vi "Illini Hyperloop GUI v3.2.vi"() -> ()   [LabVIEW 2015]
uses:
  <vilib>/robotics/Controls/Attitude Indicator/Attitude Indicator.xctl
  CommunicationStatus.ctl
  StageEnum.ctl
  BlockDiagramControlEnum.ctl
panel:
  out "Braking Force":dbl
  out "Braking Force Chart":dbl(slide) caption="Braking Force (N)" scale=0.0..10000.0
  out "Current 6":dbl[unit] caption="Current"
  out "Voltage 6":dbl[unit] caption="Voltage"
  out "RPM 6":dbl[unit] caption="RPM"
  out "Current 5":dbl[unit] caption="Current"
  out "Voltage 5":dbl[unit] caption="Voltage"
  out "RPM 5":dbl[unit] caption="RPM"
  out "Current 4":dbl[unit] caption="Current"
  out "Voltage 4":dbl[unit] caption="Voltage"
  out "RPM 4":dbl[unit] caption="RPM"
  out "Current 3":dbl[unit] caption="Current"
  out "Voltage 3":dbl[unit] caption="Voltage"
  out "RPM 3":dbl[unit] caption="RPM"
  out "Current 2":dbl[unit] caption="Current"
  out "Voltage 2":dbl[unit] caption="Voltage"
  out "RPM 2":dbl[unit] caption="RPM"
  out "Current 1":dbl[unit] caption="Current"
  out "Voltage 1":dbl[unit] caption="Voltage"
  out "RPM 1":dbl[unit] caption="RPM"
  out "Flight Time":string
  out "Attitude Indicator":cluster{"Roll":dbl, "Pitch":dbl}(xcontrol)
  out "Yaw":dbl(knob) scale=-20.0..20.0
  out "RPM Gauge 6":dbl(knob) scale=0.0..2000.0
  out "RPM Gauge 5":dbl(knob) scale=0.0..2000.0
  out "RPM Gauge 4":dbl(knob) scale=0.0..2000.0
  out "RPM Gauge 3":dbl(knob) scale=0.0..2000.0
  out "RPM Gauge 2":dbl(knob) scale=0.0..2000.0
  out "RPM Gauge 1":dbl(knob) scale=0.0..2000.0
  out "Cabin Pressure":dbl format="%#.3g"
  out "Cabin Pressure (psi)":dbl(graph)
  out "Stage":T1
  out "Communication Status":T2
  out "Levitation Height":dbl[unit]
  out "Computing:":dbl format="%#.2g"
  out "Low Battery":dbl format="%#.2g"
  out "High Battery:":dbl format="%#.2g"
  out "Battery 3":dbl(slide) scale=0.0..100.0
  out "Battery 2":dbl(slide) scale=0.0..100.0
  out "Battery 1":dbl(slide) scale=0.0..100.0
  out "Z acceleration":dbl
  out "Y acceleration":dbl
  out "X acceleration":dbl
  out "Z velocity":dbl
  out "Y velocity":dbl
  out "X velocity":dbl
  out "Z position":dbl
  out "Y position":dbl
  out "X position":dbl
  out "Position (m)":dbl(slide) scale=0.0..2490.0
  out "Velocity (m/s)":dbl(graph)
  in  "EMERGENCY BRAKE":bool
  in  "Functional Test Tab Control":T3(tab)
  out "Functional Test A Data":string caption="Data:"
  in  "Functional Test 1":bool caption="Boolean"
  out "Functional Test B Data":string caption="Data:"
  in  "Functional Test 2":bool caption="Boolean"
  out "Functional Test C Data":string caption="Data:"
  in  "Functional Test 3":bool caption="Boolean"
  in  "Functional Test 4":bool caption="Boolean"
  out "Functional Test D Data":string caption="Data:"
  out "Client Closed":string="The client VI closed the connection."
  out "Data out":string
  out "remote address":string
  out "remote port":u16
  in  "Connect to":string="192.168.137.10"
  in  "timeout ms":i32=25000
  in  "port":u16=5005
  in  "Prepare for Launch":bool caption="Boolean"
  in  "Stop Program":bool
  out "Error Messages":errorcluster
  out "Temp 2:":dbl format="%.2g"
  out "Temp 1:":dbl format="%.2g"
  out "Temperature (K)":dbl[](graph)
  out "Acceleration Chart":dbl(graph)
  out "Checkmark":u16(ring)
  # "Illini Hyperloop"
  # "Arx Pax"
  # "Front"
  # "Attitude"
  # "Acceleration (m/s/s)"
  # "Battery Levels (%)"
  # "More battery?????"
  # "Functional Test A: Power Up and Communication"
  # "Functional Test B: Levitation"
  # "Functional Test C: Communication Inside Tube"
  # "Functional Test D: Internal power and Levitation"
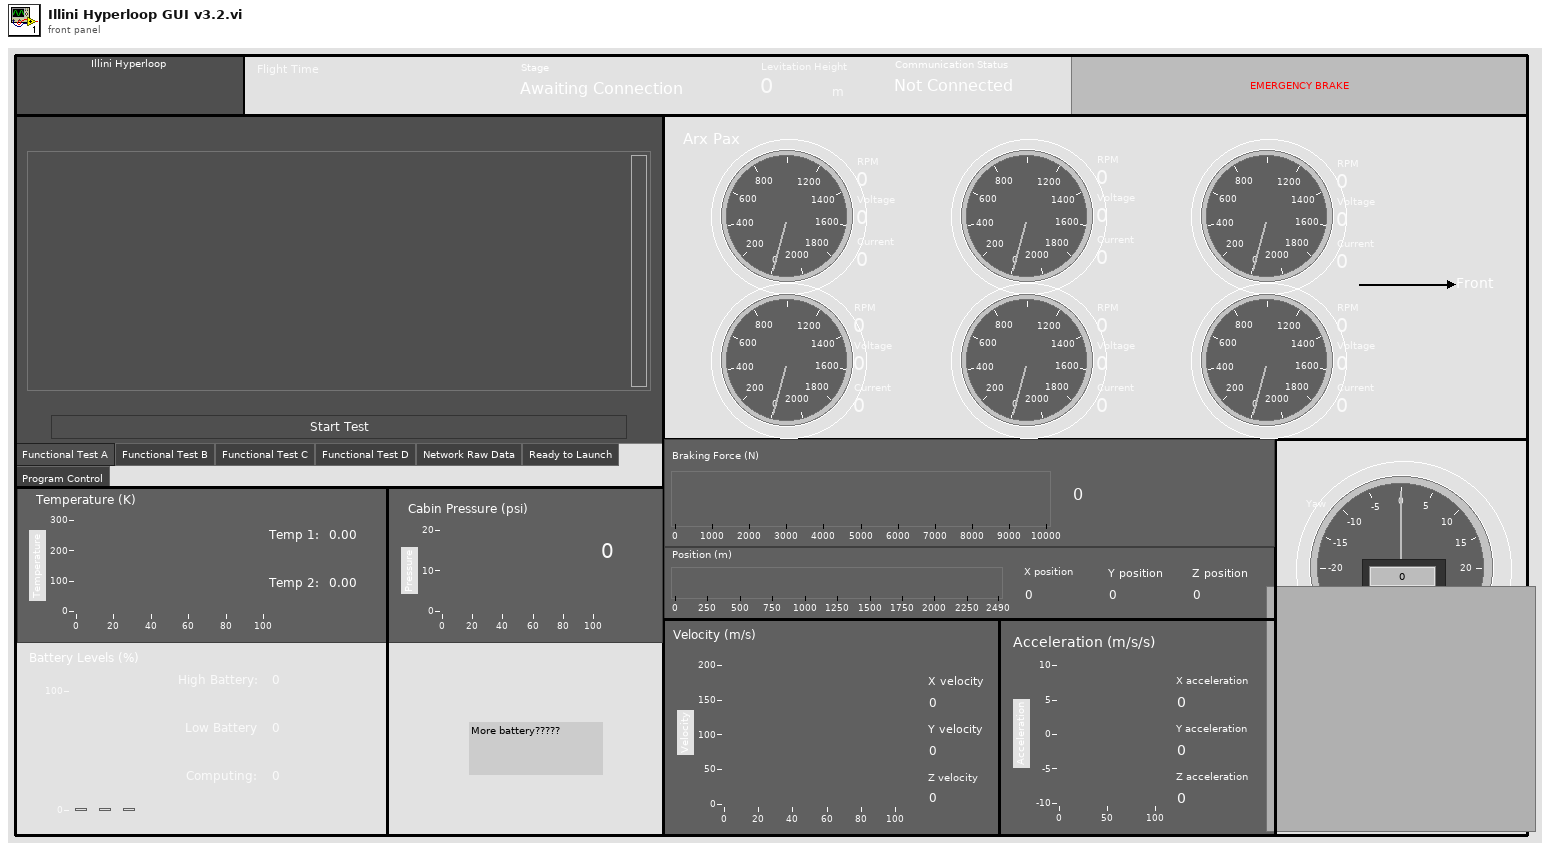
[diagram p1: front panel]
types:
  T1 = typedef "StageEnum.ctl" = enum16{"Awaiting Connection", "TEST Comms", "TEST Lev", "TEST Inside Comms", "TEST Internal Power", "Ready to Launch", "Acceleration", "Coast", "Brake"}
  T2 = typedef "CommunicationStatus.ctl" = enum16{"Not Connected", "Connected", "Disconnected"}
  T3 = enum32{"Functional Test A", "Functional Test B", "Functional Test C", "Functional Test D", "Network Raw Data", "Ready to Launch", "Program Control"}
  T4 = typedef "BlockDiagramControlEnum.ctl" = enum16{"Not Connected", "Disconnected", "Functional Test A", "Functional Test B", "Functional Test C", "Functional Test D", "Flight"}
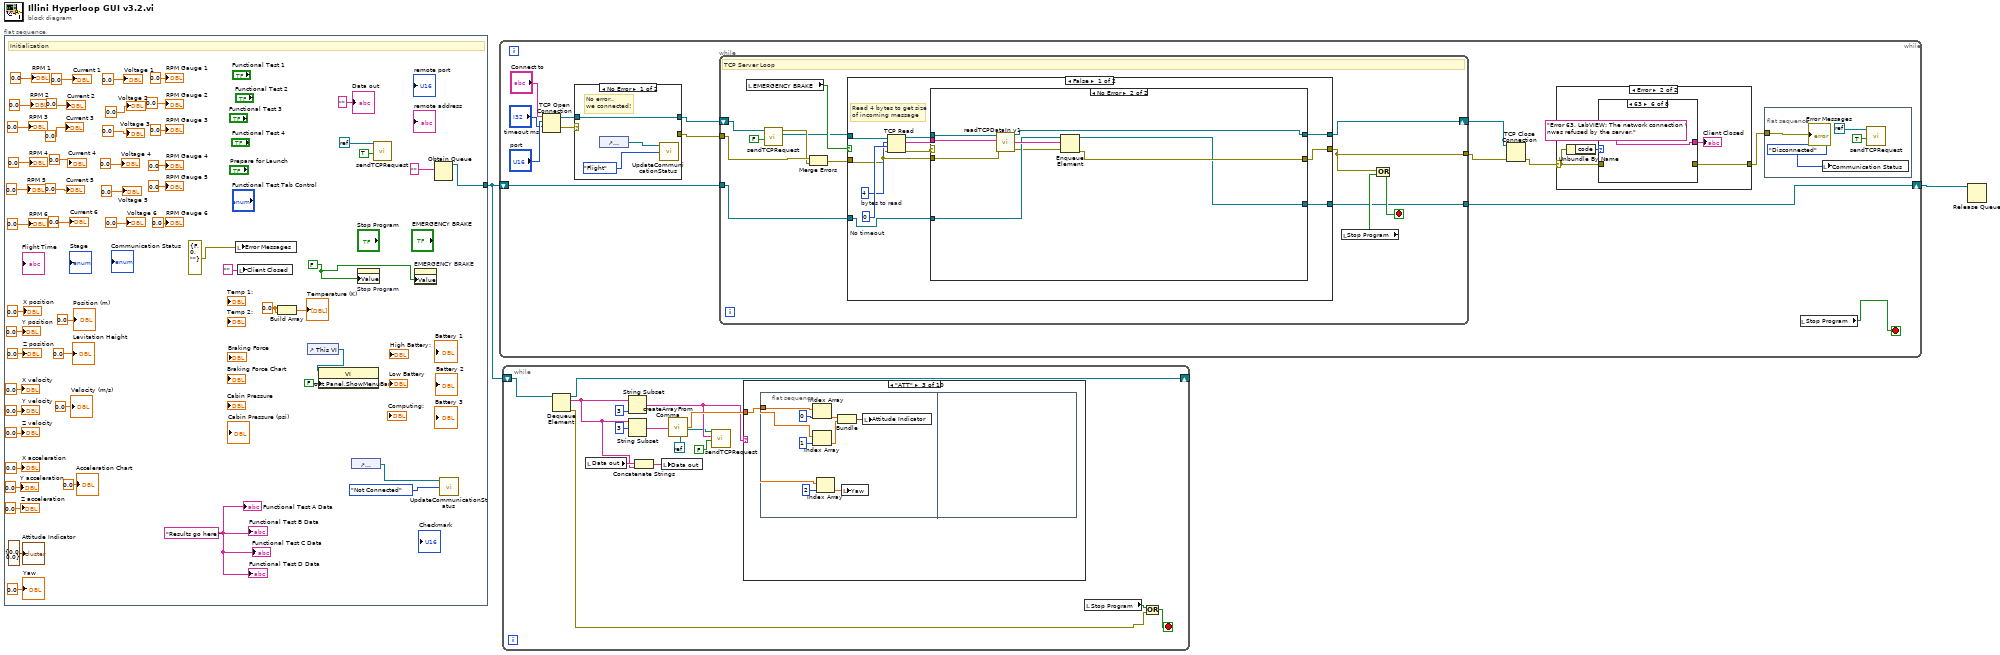
[diagram p0: block diagram]
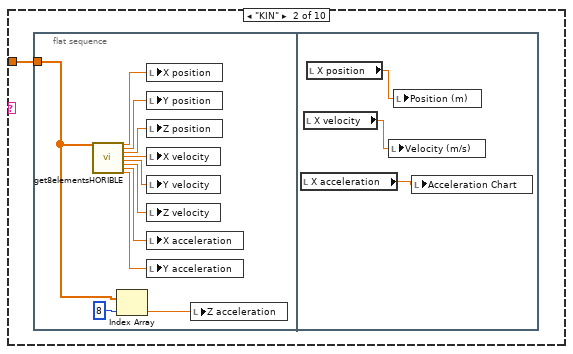
[diagram p3: hidden frame]
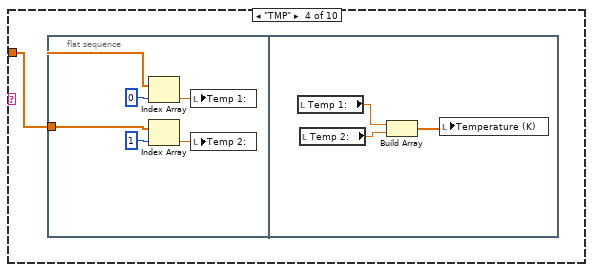
[diagram p4: hidden frame]
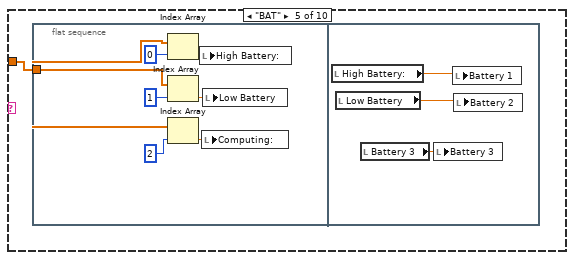
[diagram p5: hidden frame]
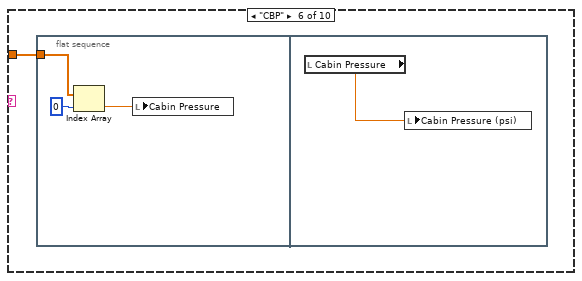
[diagram p6: hidden frame]
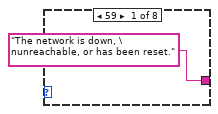
[diagram p13: hidden frame]
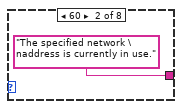
[diagram p14: hidden frame]
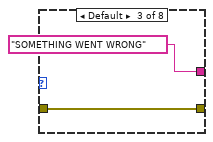
[diagram p15: hidden frame]
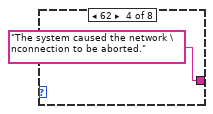
[diagram p16: hidden frame]
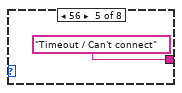
[diagram p17: hidden frame]
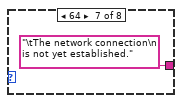
[diagram p18: hidden frame]
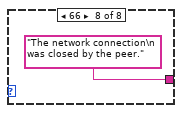
[diagram p19: hidden frame]
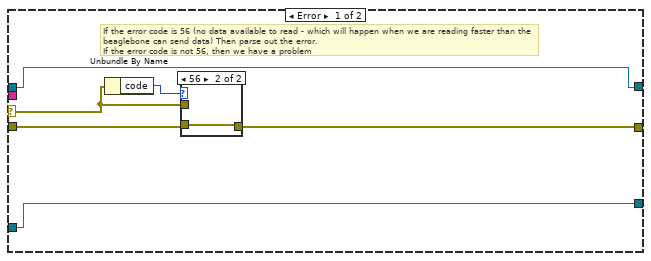
[diagram p20: hidden frame]
diagram:
  n1 = flat-sequence {
    tunnel: [w54] -> w2
    frame #0 {
      w9 = FALSE
      w14 = "Results go here!" ("Functional Test 1 Data")
      w29 = 0.0 ("element")
      # "Initialization"
      n2 = local write "Error Messages"(errorcluster {"status"=FALSE, "code"=0, "source"=""} ("error constant")) -> ()
      n3 = local write "Client Closed"("" ("Client Closed")) -> ()
      n4 = Build Array(w29, w29) -> (→"Temperature (K)":dbl[])
      n5 = control-ref of="This VI"() -> (w8:refnum<vi>)
      n6 = property class="VI"(reference=w8, "Front Panel.ShowMenuBar"=FALSE ("Front Panel Window:Show Menu Bar")) -> ()  [unwired: 1 in, 2 out]
      n7 = control-ref of="Communication Status"() -> (w56:refnum<vi>)
      n8 = property on="Stop Program" class="Bool (strict)"("Value"=w9) -> ()  [unwired: 2 in, 2 out]
      n9 = call "sendTCPRequest.vi"("Force Reset"=TRUE, "TCP Network Connection in"=refnum<k0> refnum) -> ()  [unwired: 8 in, 2 out]
      n10 = property on="EMERGENCY BRAKE" class="Bool (strict)"("Value"=w9) -> ()  [unwired: 2 in, 2 out]
      n11 = Obtain Queue(element data type="") -> (queue out=w54:refnum<queue>)  [unwired: 4 in, 2 out]
      n12 = call "UpdateCommunicationStatus.vi"("Block Diagram Control Enum"=BlockDiagramControlEnum."Not Connected", "Communication Enum Refnum in"=w56) -> ()  [unwired: 1 in]
      "RPM Gauge 2" <- 0.0 ("RPM Gauge 2")
      "RPM Gauge 4" <- 0.0 ("RPM Gauge 4")
      "RPM Gauge 5" <- 0.0 ("RPM Gauge 5")
      "RPM Gauge 1" <- 0.0 ("RPM Gauge 1")
      "RPM Gauge 6" <- 0.0 ("RPM Gauge 6")
      "RPM Gauge 3" <- 0.0 ("RPM Gauge 3")
      "RPM 1" <- dbl[unit] 0.0 ("RPM 1")
      "Current 1" <- dbl[unit] 0.0 ("Current 1")
      "RPM 2" <- dbl[unit] 0.0 ("RPM 2")
      "Voltage 2" <- dbl[unit] 0.0 ("Voltage 2")
      "Current 2" <- dbl[unit] 0.0 ("Current 2")
      "RPM 3" <- dbl[unit] 0.0 ("RPM 3")
      "Voltage 3" <- dbl[unit] 0.0 ("Voltage 3")
      "Current 3" <- dbl[unit] 0.0 ("Current 3")
      "RPM 4" <- dbl[unit] 0.0 ("RPM 4")
      "Voltage 4" <- dbl[unit] 0.0 ("Voltage 4")
      "Current 4" <- dbl[unit] 0.0 ("Current 4")
      "RPM 5" <- dbl[unit] 0.0 ("RPM 5")
      "Voltage 5" <- dbl[unit] 0.0 ("Voltage 5")
      "Current 5" <- dbl[unit] 0.0 ("Current 5")
      "RPM 6" <- dbl[unit] 0.0 ("RPM 6")
      "Voltage 6" <- dbl[unit] 0.0 ("Voltage 6")
      "Current 6" <- dbl[unit] 0.0 ("Current 6")
      "Voltage 1" <- dbl[unit] 0.0 ("Voltage 1")
      "Position (m)" <- 0.0 ("Position (m)")
      "X position" <- 0.0 ("X position")
      "Y position" <- 0.0 ("Y position")
      "Z position" <- 0.0 ("Z position")
      "X velocity" <- 0.0 ("X velocity")
      "Y velocity" <- 0.0 ("Y velocity")
      "Z velocity" <- 0.0 ("Z velocity")
      "X acceleration" <- 0.0 ("X acceleration")
      "Y acceleration" <- 0.0 ("Y acceleration")
      "Z acceleration" <- 0.0 ("Z acceleration")
      "Velocity (m/s)" <- 0.0 ("Velocity (m/s)")
      "Attitude Indicator" <- cluster{"Roll":dbl, "Pitch":dbl} {"Roll"=0.0, "Pitch"=0.0} ("Attitude Indicator")
      "Levitation Height" <- dbl[unit] 0.0 ("Levitation Height")
      "Acceleration Chart" <- 0.0 ("Acceleration Chart")
      "Yaw" <- 0.0 ("Yaw")
      "Functional Test A Data" <- w14
      "Functional Test B Data" <- w14
      "Functional Test C Data" <- w14
      "Functional Test D Data" <- w14
      "Data out" <- "" ("Data out")
    }
  }
  n13 = while {
    shift-right: [w63] -> w1
    shift-left: w2 -> [w64]
    stop <- w60 stop-if-true
    n14 = TCP Open Connection(address="Connect to", remote port or service name="port", timeout ms (60000)="timeout ms") -> (connection ID=w65:refnum<k5>, error out=w66:errorcluster)  [unwired: 2 in]
    n15 = case shown="No Error" w66 {
      selector: w66 -> [_ w78]
      tunnel: w65 -> [w77 w79]
      tunnel: [w77 w79] -> w58
      tunnel: [_ w78] -> w57
      frame No Error {
        # "No error.. \nwe connected!"
        n16 = control-ref of="Communication Status"() -> (w76:refnum<vi>)
        n17 = call "UpdateCommunicationStatus.vi"("Block Diagram Control Enum"=BlockDiagramControlEnum."Flight", "Communication Enum Refnum in"=w76) -> ()  [unwired: 1 in]
      }
      frame Error {
      }
    }
    n18 = while {
      tunnel: w57 -> [w98]
      tunnel: [w104] -> w62
      tunnel: w64 -> [w102]
      tunnel: [w101] -> w63
      shift-right: [w100] -> w59
      shift-left: w58 -> [w99]
      stop <- w103 stop-if-true
      # "TCP Server Loop"
      n19 = local read "EMERGENCY BRAKE"() -> (w106:bool)
      n20 = call "sendTCPRequest.vi"("Force Reset"=FALSE, "TCP Network Connection in"=w99) -> ("Connection Out"=w96:refnum<k5>, "error out"=w97:errorcluster)  [unwired: 8 in]
      n21 = Merge Errors(w98, w97) -> (w94:errorcluster)
      n22 = case shown="False" w106 {
        tunnel: w94 -> [w115 w140]
        tunnel: w96 -> [w116 w139]
        tunnel: [w112 w138] -> w100
        tunnel: [w108 w137] -> w104
        tunnel: w102 -> [w110 w136]
        tunnel: [w109 w136] -> w101
        frame False {
          w117 = 4  # bytes to read
          w118 = 0  # No timeout
          # "Read 4 bytes to get size\nof incoming message"
          n23 = TCP Read(connection ID=w116, bytes to read=w117, error in (no error)=w115, 9:w118) -> (connection ID out=w113:refnum<k5>, data out=w111:string, error out=w114:errorcluster)  [unwired: 1 in]
          n24 = case shown="No Error" w114 {
            selector: w114 -> [w122 _]
            tunnel: w115 -> [w123 w133]
            tunnel: [w121 w128] -> w108
            tunnel: w113 -> [w120 w134]
            tunnel: [w120 w132] -> w112
            tunnel: w111 -> [_ w135]
            tunnel: w110 -> [w119 w130]
            tunnel: [w119 w127] -> w109
            frame Error {
              # "If the error code is 56 (no data available to read - which will happen when we are reading faster than the beaglebone can send data) Then parse out the error. \nIf the error code is not 56, then we have a problem"
              n25 = Unbundle By Name(w122) -> ("code"=w124:i32)
              n26 = case shown="56" w124 {
                tunnel: w122 -> [w125 _]
                tunnel: [w125 w126] -> w121
                tunnel: w123 -> [_ w126]
                frame Default {
                }
                frame 56 {
                }
              }
            }
            frame No Error {
              n27 = call "readTCPDataIn v1.vi"("TCP Network Connection in"=w134, "Size of data"=w135, "error in (no error)"=w133) -> ("TCP Network Connection out"=w132:refnum<k5>, "Operation+Data"=w131:string, "error out"=w129:errorcluster)  [unwired: 8 in, 2 out]
              n28 = Enqueue Element(queue=w130, element=w131, error in (no error)=w129) -> (queue out=w127:refnum<queue>, error out=w128:errorcluster)  [unwired: 1 in, 1 out]
            }
          }
        }
        frame True {
          n29 = TCP Write(connection ID=w139, data in="STOP!STOP", error in (no error)=w140) -> (connection ID out=w138:refnum<k5>, error out=w137:errorcluster)  [unwired: 1 in, 1 out]
        }
      }
      n30 = local read "Stop Program"() -> (w105:bool)
      n31 = Or(x=w104, y=w105) -> (x .or. y?=w103:bool)
      n32 = Wait (ms)(milliseconds to wait=u32 0) -> ()  [unwired: 1 out]
    }
    n33 = TCP Close Connection(connection ID=w59, error in (no error)=w62) -> (error out=w70:errorcluster)  [unwired: 2 out]
    n34 = case shown="Error" w70 {
      selector: w70 -> [w80 w83]
      tunnel: [w80 w82] -> w69
      frame No Error {
      }
      frame Error {
        n35 = Unbundle By Name(w83) -> ("code"=w84:i32)
        n36 = case shown="63" w84 {
          tunnel: w83 -> [_ _ w88 _ _ _ _ _]
          tunnel: [_ _ w88 _ _ _ _ _] -> w82
          tunnel: ["The network is down, \nunreachable, or has been reset." "The specified network \naddress is currently in use." "SOMETHING WENT WRONG" "The system caused the network \nconnection to be aborted." "Timeout / Can't connect" "Error 63. LabVIEW: The network connection \nwas refused by the server." "\tThe network connection\n is not yet established." "The network connection\n was closed by the peer."] -> w81
          frame 59 {
          }
          frame 60 {
          }
          frame Default {
          }
          frame 62 {
          }
          frame 56 {
          }
          frame 63 {
          }
          frame 64 {
          }
          frame 66 {
          }
        }
        "Client Closed" <- w81
      }
    }
    n37 = flat-sequence {
      tunnel: w69 -> [w74]
      frame #0 {
        n38 = local write "Communication Status"(CommunicationStatus."Disconnected" ("Communication Status")) -> ()
        n39 = call "sendTCPRequest.vi"("Force Reset"=TRUE, "TCP Network Connection in"=refnum<k0> refnum) -> ()  [unwired: 8 in, 2 out]
        "Error Messages" <- w74
      }
    }
    n40 = local read "Stop Program"() -> (w60:bool)
  }
  n41 = while {
    shift-right: [w156] -> _
    shift-left: w2 -> [w151]
    stop <- w145 stop-if-true
    n42 = Dequeue Element(queue=w151) -> (queue out=w156:refnum<queue>, element=w149:string, error out=w146:errorcluster)  [unwired: 2 in, 1 out]
    n43 = local read "Data out"() -> (w150:string)
    n44 = String Subset(string=w149, length (rest)=3 ("length (rest)")) -> (substring=w144:string)  [unwired: 1 in]
    n45 = String Subset(string=w149, offset (0)=3) -> (substring=w153:string)  [unwired: 1 in]
    n46 = Concatenate Strings(w150, w149) -> (w148:string)
    n47 = local write "Data out"(w148) -> ()
    n48 = call "createArrayFromComma.vi"("String"=w153) -> ("Array"=w152:dbl[])
    n49 = call "sendTCPRequest.vi"("Force Reset"=FALSE, "String"=w144, "TCP Network Connection in"=refnum<k0> refnum) -> ()  [unwired: 7 in, 2 out]
    n50 = case shown="\"ATT\"" w144 {
      tunnel: w152 -> [_ w157 w172 w181 w190 w201 _ _ _ _]
      frame Default {
      }
      frame "KIN" {
        n51 = flat-sequence {
          tunnel: w157 -> [w167]
          frame #0 {
            n52 = call "get8elementsHORIBLE.vi"("Array"=w167) -> ("Numeric"=w165:dbl, "Numeric 2"=w164:dbl, "Numeric 3"=w163:dbl, "Numeric 4"=w162:dbl, "Numeric 5"=w161:dbl, "Numeric 6"=w160:dbl, "Numeric 7"=w159:dbl, "Numeric 8"=w158:dbl)  [unwired: 19 in]
            n53 = Index Array(array=w167, index=8) -> (element=w166:dbl)
            n54 = local write "X position"(w165) -> ()
            n55 = local write "Y position"(w164) -> ()
            n56 = local write "Z position"(w163) -> ()
            n57 = local write "X velocity"(w162) -> ()
            n58 = local write "Y velocity"(w161) -> ()
            n59 = local write "Z velocity"(w160) -> ()
            n60 = local write "X acceleration"(w159) -> ()
            n61 = local write "Y acceleration"(w158) -> ()
            n62 = local write "Z acceleration"(w166) -> ()
          }
          frame #1 {
            n63 = local read "X acceleration"() -> (w171:dbl)
            n64 = local read "X velocity"() -> (w170:dbl)
            n65 = local read "X position"() -> (w169:dbl)
            n66 = local write "Velocity (m/s)"(w170) -> ()
            n67 = local write "Position (m)"(w169) -> ()
            n68 = local write "Acceleration Chart"(w171) -> ()
          }
        }
      }
      frame "ATT" {
        n69 = flat-sequence {
          tunnel: w172 -> [w177]
          frame #0 {
            n70 = Index Array(array=w177, index=0) -> (element=w176:dbl)
            n71 = Index Array(array=w177, index=1) -> (element=w175:dbl)
            n72 = Index Array(array=w177, index=2) -> (element=w173:dbl)
            n73 = Bundle(w176, w175) -> (w174:cluster{dbl, dbl})  [unwired: 1 in]
            n74 = local write "Yaw"(w173) -> ()
            n75 = local write "Attitude Indicator"(w174) -> ()
          }
          frame #1 {
          }
        }
      }
      frame "TMP" {
        n76 = flat-sequence {
          tunnel: w181 -> [w184]
          frame #0 {
            n77 = Index Array(array=w184, index=0) -> (element=w183:dbl)
            n78 = Index Array(array=w184, index=1) -> (element=w182:dbl)
            n79 = local write "Temp 1:"(w183) -> ()
            n80 = local write "Temp 2:"(w182) -> ()
          }
          frame #1 {
            n81 = local read "Temp 1:"() -> (w187:dbl)
            n82 = local read "Temp 2:"() -> (w188:dbl)
            n83 = Build Array(w187, w188) -> (w189:dbl[])
            n84 = local write "Temperature (K)"(w189) -> ()
          }
        }
      }
      frame "BAT" {
        n85 = flat-sequence {
          tunnel: w190 -> [w194]
          frame #0 {
            n86 = Index Array(array=w194, index=0) -> (element=w193:dbl)
            n87 = Index Array(array=w194, index=1) -> (element=w192:dbl)
            n88 = Index Array(array=w194, index=2) -> (element=w191:dbl)
            n89 = local write "High Battery:"(w193) -> ()
            n90 = local write "Computing:"(w191) -> ()
            n91 = local write "Low Battery"(w192) -> ()
          }
          frame #1 {
            n92 = local read "High Battery:"() -> (w199:dbl)
            n93 = local read "Low Battery"() -> (w200:dbl)
            n94 = local read "Battery 3"() -> (w198:dbl)
            n95 = local write "Battery 3"(w198) -> ()
            n96 = local write "Battery 1"(w199) -> ()
            n97 = local write "Battery 2"(w200) -> ()
          }
        }
      }
      frame "CBP" {
        n98 = flat-sequence {
          tunnel: w201 -> [w203]
          frame #0 {
            n99 = Index Array(array=w203, index=0) -> (element=w202:dbl)
            n100 = local write "Cabin Pressure"(w202) -> ()
          }
          frame #1 {
            n101 = local read "Cabin Pressure"() -> (w205:dbl)
            n102 = local write "Cabin Pressure (psi)"(w205) -> ()
          }
        }
      }
      frame "FTA" {
      }
      frame "FTB" {
      }
      frame "FCC" {
      }
      frame "FCD" {
      }
    }
    n103 = local read "Stop Program"() -> (w147:bool)
    n104 = Or(x=w147, y=w146) -> (x .or. y?=w145:bool)
  }
  n105 = Release Queue(queue=w1) -> ()  [unwired: 2 in, 3 out]
